vi "TX Message.vi"(8 "error in (no error)":errorcluster, 10 "variant":variant, 11 "Engine RPM in":refnum<class "Engine RPM.lvclass">) -> (0 "error out":errorcluster, 3 "Engine RPM out":refnum<class "Engine RPM.lvclass">)   [LabVIEW 2011, in "Engine RPM.lvclass"]
uses:
  Engine RPM.lvclass
  PID.lvclass
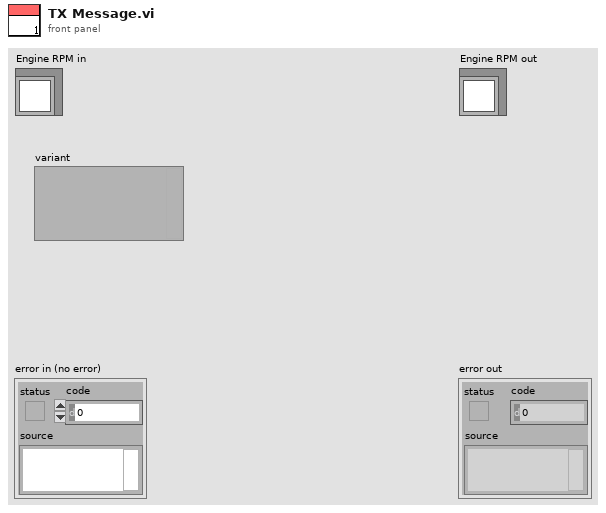
[diagram p1: front panel]
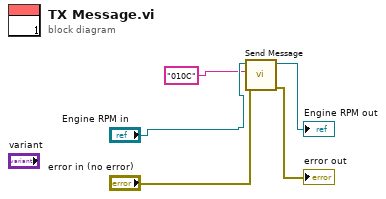
[diagram p0: block diagram]
diagram:
  n1 = call "Send Message.vi"("error in (no error)"="error in (no error)", "TX Message"="010C", "PID in"="Engine RPM in") -> ("error out"=→"error out":errorcluster, "PID out"=→"Engine RPM out":refnum<class "Engine RPM.lvclass">)  [unwired: 7 in]
